vi "Stop ADB Server.vi"(0 "adb location":string, 1 "error in":errorcluster) -> (4 "error out":errorcluster)   [LabVIEW 2016]
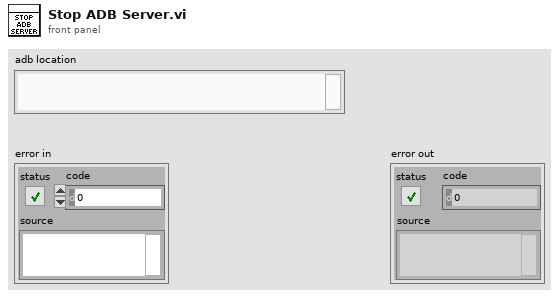
[diagram p1: front panel]
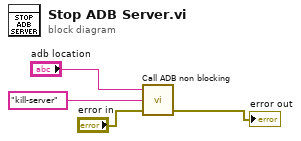
[diagram p0: block diagram]
diagram:
  n1 = call "Call ADB non blocking.vi"("error in"="error in", "adb sub-command"="kill-server", "adb location"="adb location") -> ("error out"=→"error out":errorcluster)  [unwired: 2 in]
